vi "IGC100.vi"(8 "IGC100 B Error":refnum<vi>, 9 "IGC100 A Error":refnum<vi>, 11 "QUIT":refnum<vi>) -> ()   [LabVIEW 2018]
uses:
  <vilib>/Utility/error.llb/DialogType.ctl
  <vilib>/Analysis/baseanly.llb/Mean (DBL).vi
  <vilib>/Analysis/NI_AALBase.lvlib
panel:
  out "Main Error":errorcluster
  in  "IGC100":T1(tab)
  out "A PG1":dbl caption="PG1"
  out "A AN4":dbl caption="AN4"
  out "A AN3":dbl caption="AN3"
  out "A AN2":dbl caption="AN2"
  out "A AN1":dbl caption="AN1"
  out "A CM4":dbl caption="CM4"
  out "A CM3":dbl caption="CM3"
  out "A CM2":dbl caption="CM2"
  out "A IG2":dbl caption="IG2" format="%#_4e"
  out "A IG1":dbl caption="IG1" format="%#_4e"
  out "A PG2":dbl caption="PG2"
  out "A CM1":dbl caption="CM1"
  out "IGC100 B Status":string
  out "IGC100 A Status":string
  out "B IG1":dbl caption="IG1" format="%#2_4e"
  out "B IG2":dbl caption="IG2"
  out "B PG1":dbl caption="PG1" format="%#2_4e"
  out "B PG2":dbl caption="PG2" format="%#_4e"
  out "B AN1":dbl caption="AN1"
  out "B AN2":dbl caption="AN2"
  out "B AN3":dbl caption="AN3"
  out "B AN4":dbl caption="AN4"
  out "B CM1":dbl caption="CM1"
  out "B CM2":dbl caption="CM2"
  out "B CM3":dbl caption="CM3"
  out "B CM4":dbl caption="CM4"
  out "Logging":bool
  in  "Log Pressures":bool
  in  "Advanced Settings":bool caption="(This may take some\ntime to load.)"
  in  "Communication Interval (ms)":u32
  in  "Log Interval (s)":u32=1 min=1
  in  "Averaging Time (s)":u32=1
  in  "Enable IGC100 A":bool=TRUE
  in  "Enable IGC100 B":bool=TRUE
  out "IGC100 B Online":bool
  out "IGC100 A Online":bool
  in  "IGC100 A Port":refnum<visa-resource-name>="COM11"
  in  "IGC100 B Port":refnum<visa-resource-name>="COM9"
  out "IGC100 A error":errorcluster
  out "IGC100 B error":errorcluster
  # "IG1"
  # "IGC100 A"
  # "IGC100 B"
  # "Units are in Torr"
  # "Measurements continue after window is closed."
  # "Turn off the logging feature to save CPU power and\nhard drive space."
  # "Currenty, the first column in the log file is the time of day, in hours, expressed as a decmal.  The 24 measurements then follow in the order specified in the IGC100 manual.  First for A (12), then B (another 12).\n\nIG1, IG2, PG1,... AN4"
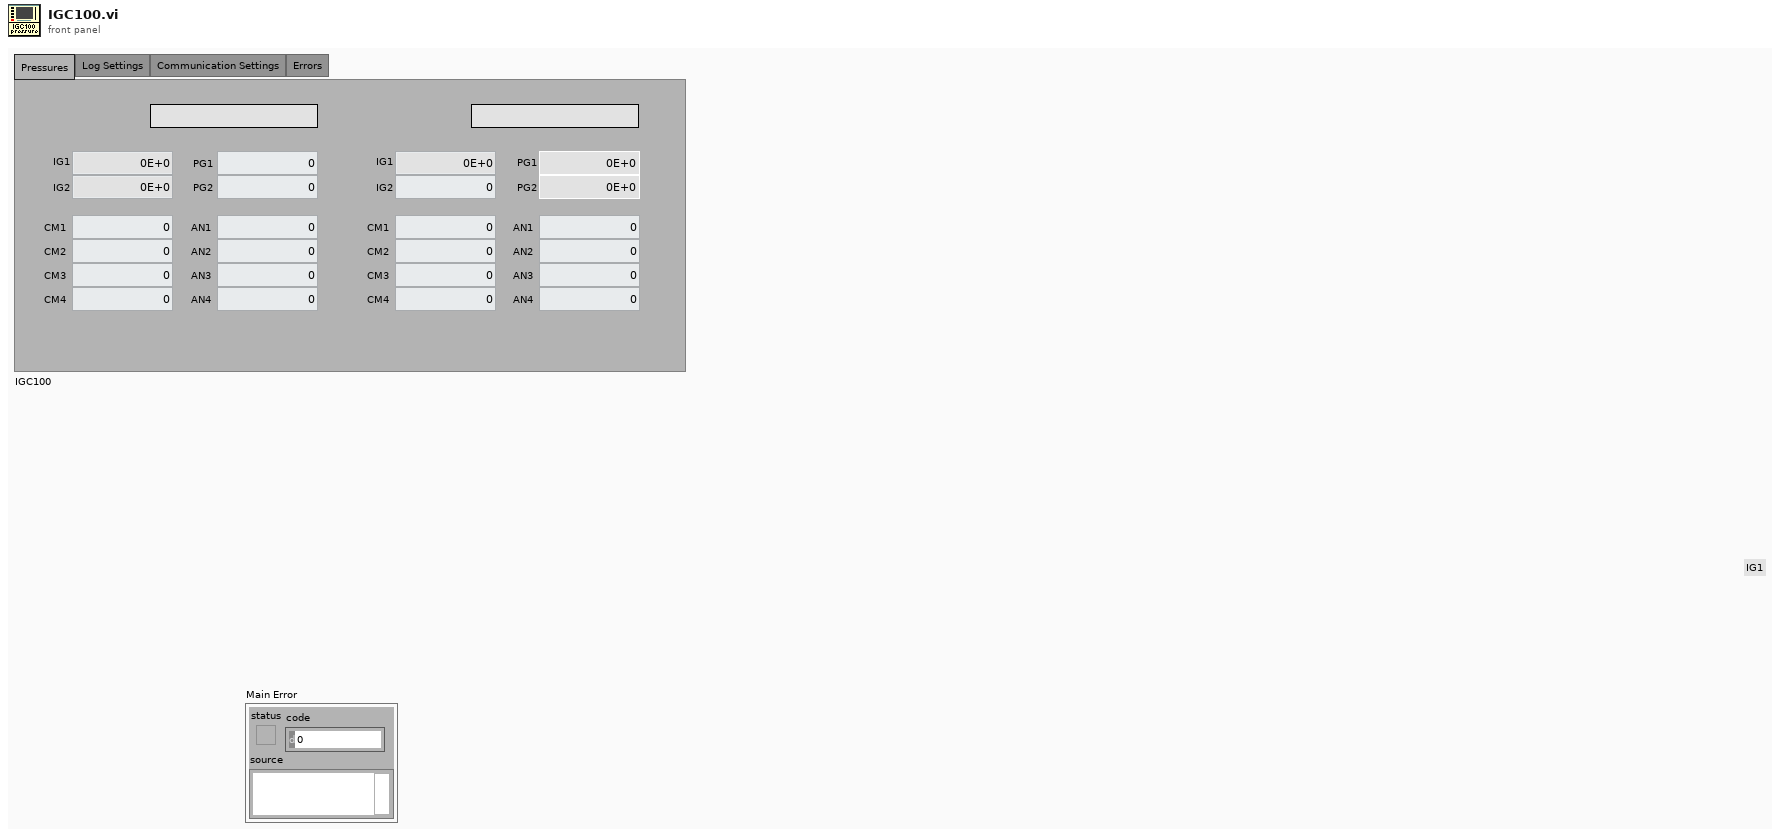
[diagram p1: front panel]
types:
  T1 = enum32{"Pressures", "Log Settings", "Communication Settings", "Errors"}
  T2 = typedef "DialogType.ctl" = u16
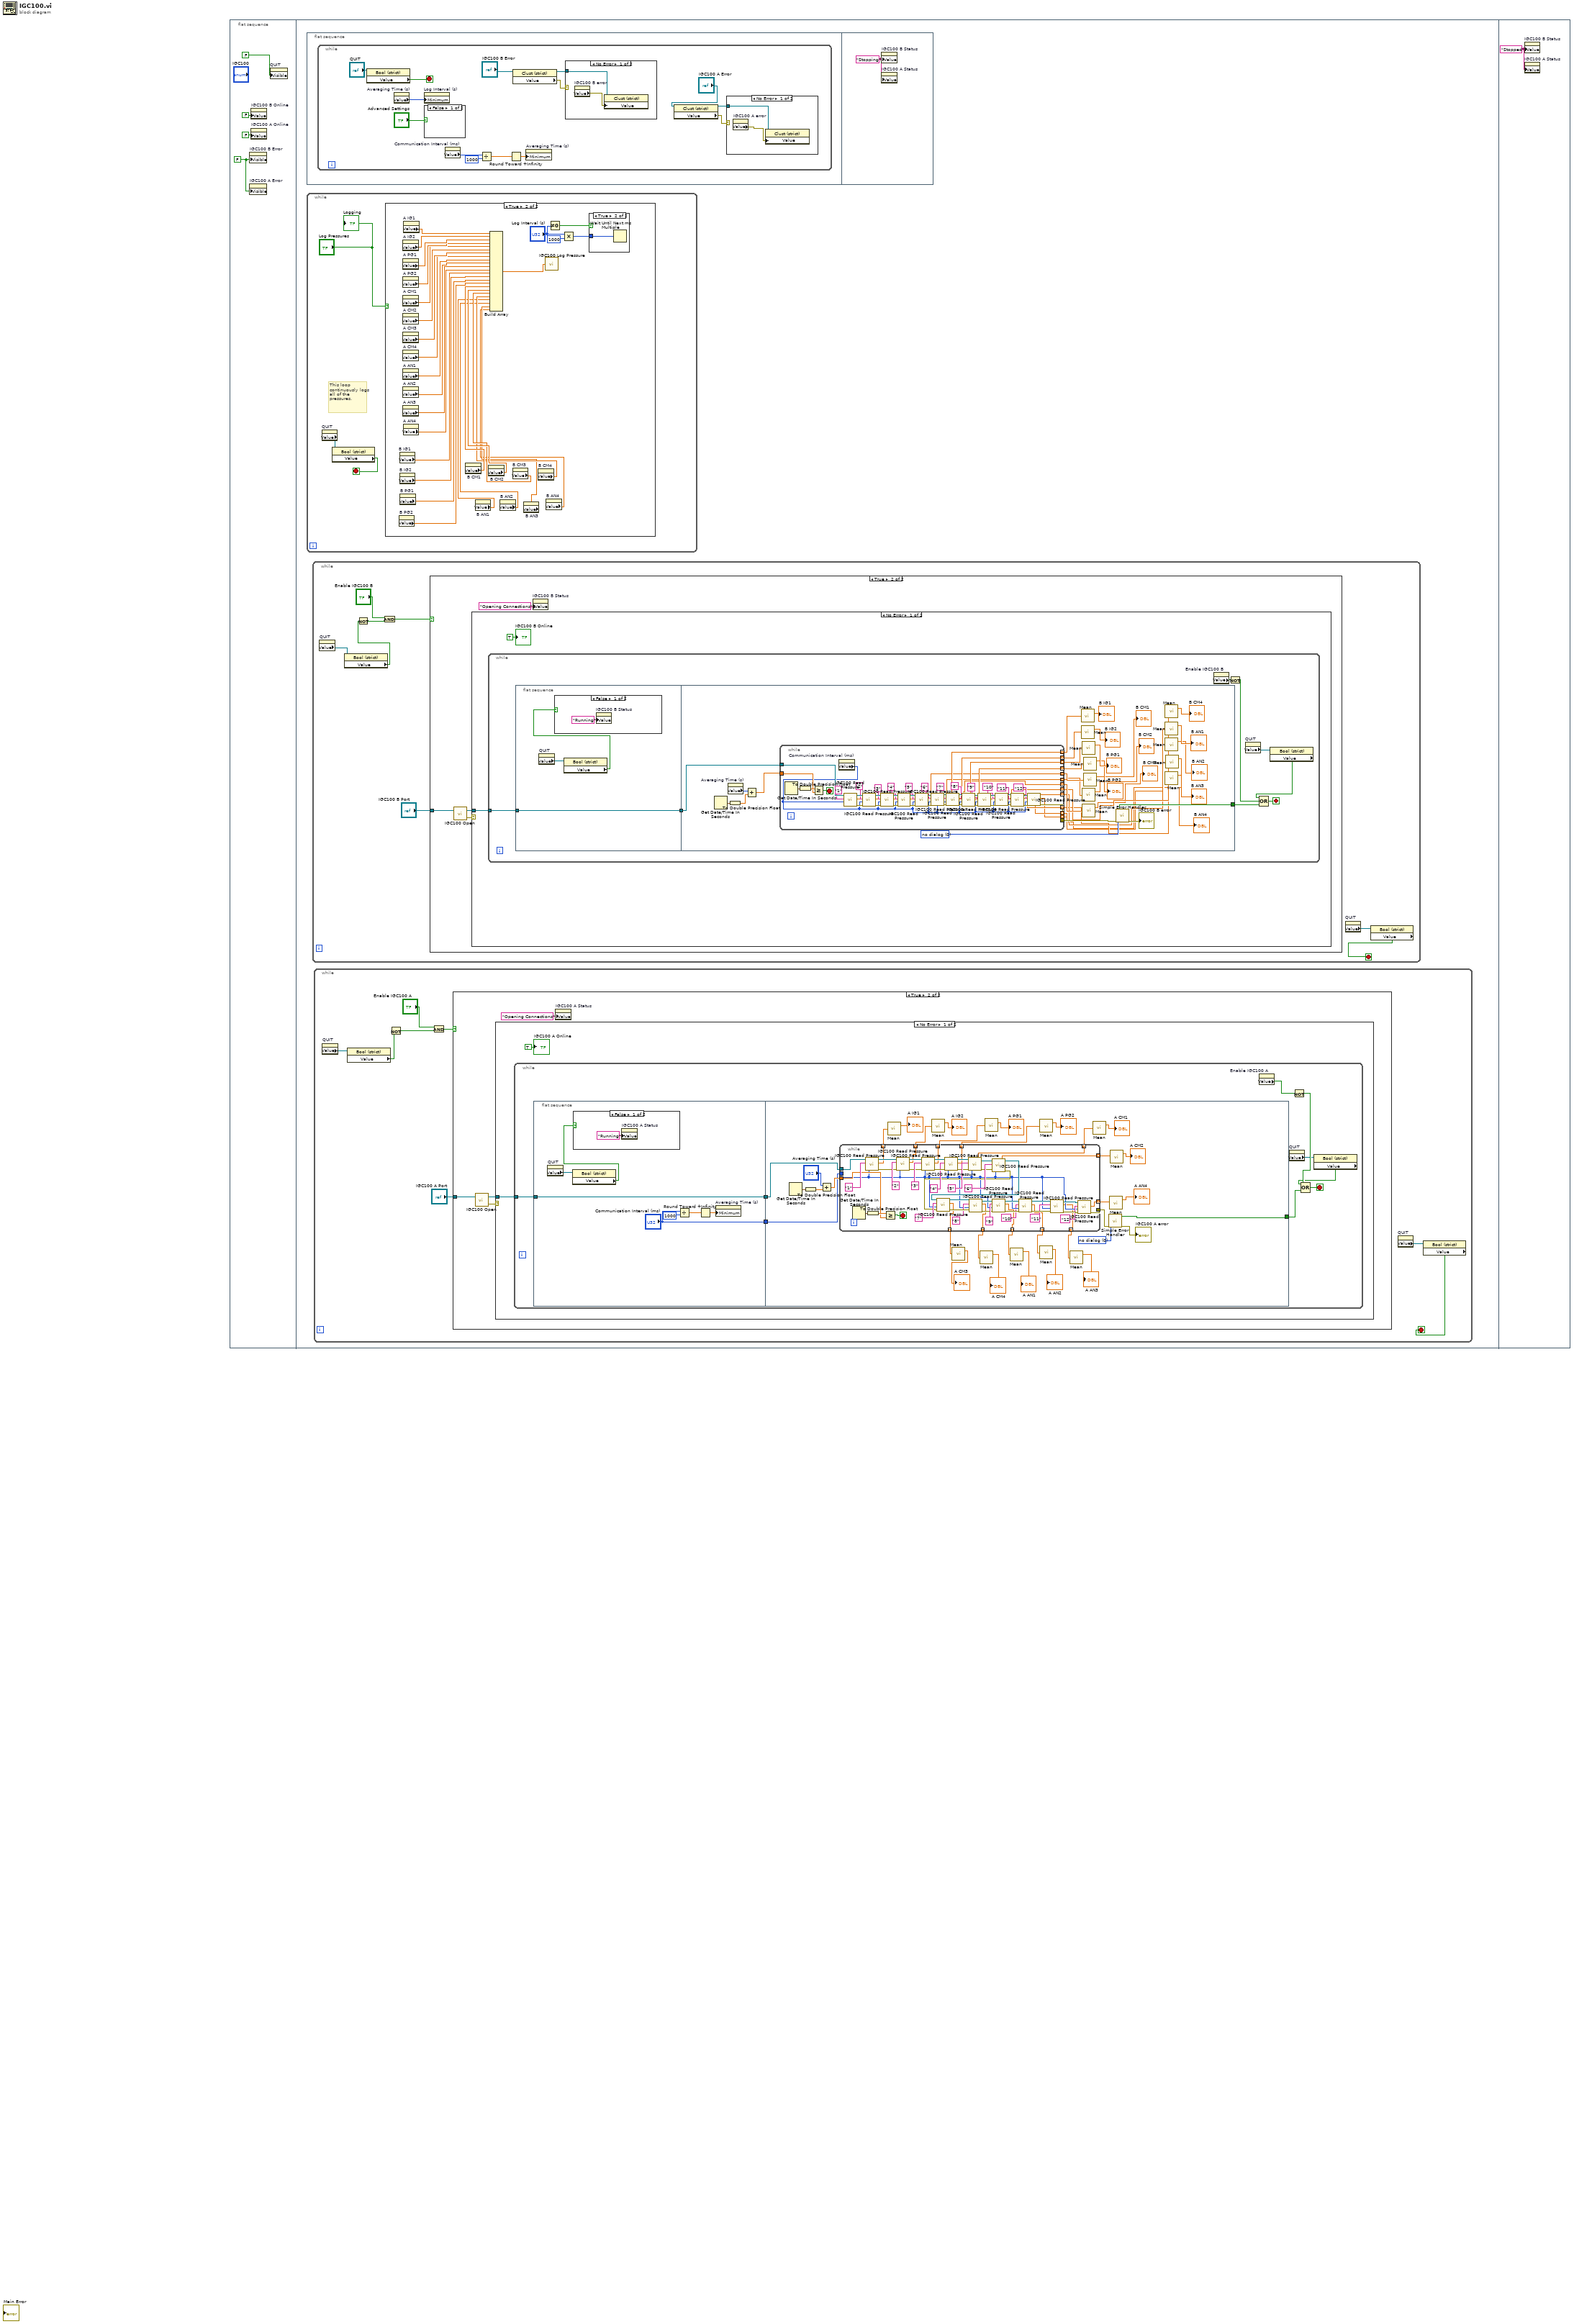
[diagram p0: block diagram]
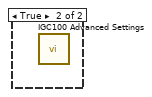
[diagram p4: hidden frame]
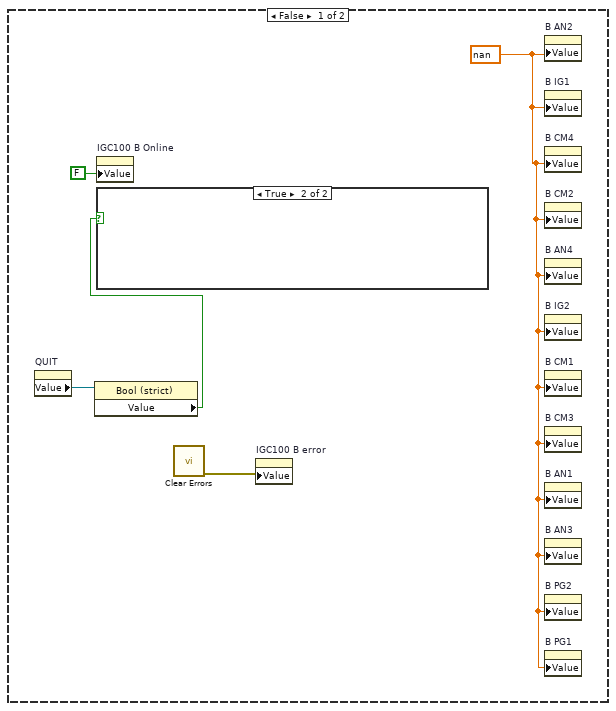
[diagram p7: hidden frame]
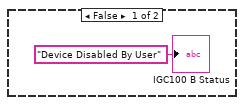
[diagram p8: hidden frame]
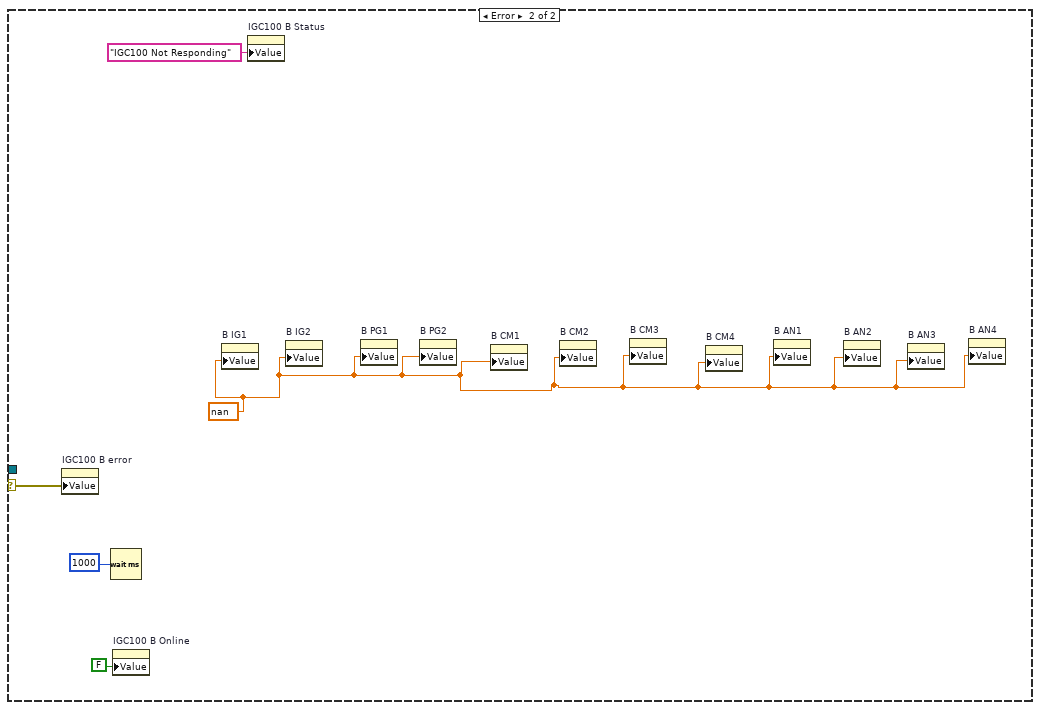
[diagram p10: hidden frame]
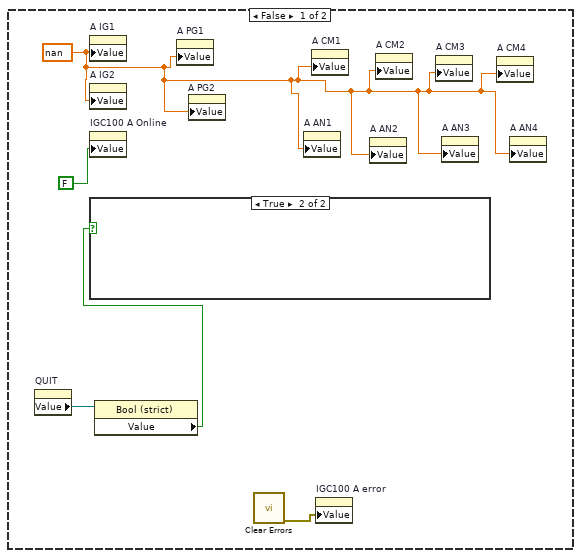
[diagram p11: hidden frame]
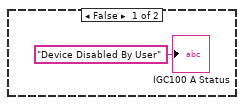
[diagram p12: hidden frame]
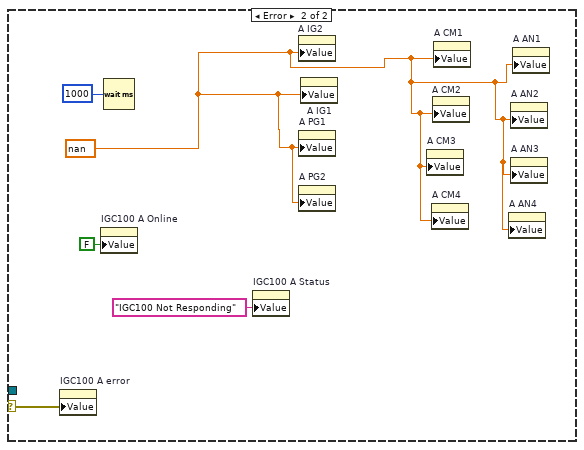
[diagram p14: hidden frame]
diagram:
  n1 = flat-sequence {
    frame #0 {
      w1 = FALSE ("Visible")
      n2 = property on="IGC100 B Error" class="LVObjRef (strict)"("Visible"=w1) -> ()  [unwired: 2 in, 2 out]
      n3 = property on="IGC100 A Error" class="LVObjRef (strict)"("Visible"=w1) -> ()  [unwired: 2 in, 2 out]
      n4 = property on="IGC100 B Online" class="Bool (strict)"("Value"=FALSE ("IGC100 Prep Online")) -> ()  [unwired: 2 in, 2 out]
      n5 = property on="IGC100 A Online" class="Bool (strict)"("Value"=FALSE ("IGC100 Main Online")) -> ()  [unwired: 2 in, 2 out]
      n6 = property on="QUIT" class="LVObjRef (strict)"("Visible"=FALSE ("QUIT")) -> ()  [unwired: 2 in, 2 out]
    }
    frame #1 {
      n7 = flat-sequence {
        frame #0 {
          n8 = while {
            stop <- w17 stop-if-true
            n9 = property on="Property Node" class="Bool (strict)"(reference="QUIT") -> ("Value"=w17:bool)  [unwired: 1 in, 2 out]
            n10 = property on="Averaging Time (s)" class="DigNum (strict)"() -> ("Value"=w12:u32)  [unwired: 2 in, 2 out]
            n11 = property on="Log Interval (s)" class="DigNum (strict)"("Minimum"=w12) -> ()  [unwired: 2 in, 2 out]
            n12 = case shown="False" "Advanced Settings" {
              frame False {
              }
              frame True {
                n13 = call "IGC100 Advanced Settings.vi"() -> ()  [unwired: 12 in]
              }
            }
            n14 = property on="Communication Interval (ms)" class="DigNum (strict)"() -> ("Value"=w14:u32)  [unwired: 2 in, 2 out]
            n15 = Divide(x=w14, y=u32 1000) -> (x/y=w15:dbl)
            n16 = Round Toward +Infinity(x=w15) -> (ceil(x): smallest int >= x=w16:dbl)
            n17 = property on="Property Node" class="Clust (strict)"(reference="IGC100 B Error") -> (reference out=w8:refnum<vi>, "Value"=w9:errorcluster)  [unwired: 1 in, 1 out]
            n18 = property on="Averaging Time (s)" class="DigNum (strict)"("Minimum"=w16) -> ()  [unwired: 2 in, 2 out]
            n19 = case shown="No Error" w9 {
              tunnel: w8 -> [w21 _]
              frame No Error {
                n20 = property on="IGC100 B error" class="Clust (strict)"() -> ("Value"=w22:errorcluster)  [unwired: 2 in, 2 out]
                n21 = property on="Property Node" class="Clust (strict)"(reference=w21, "Value"=w22) -> ()  [unwired: 1 in, 2 out]
              }
              frame Error {
              }
            }
            n22 = property on="Property Node" class="Clust (strict)"(reference="IGC100 A Error") -> (reference out=w7:refnum<vi>, "Value"=w6:errorcluster)  [unwired: 1 in, 1 out]
            n23 = case shown="No Error" w6 {
              tunnel: w7 -> [w20 _]
              frame No Error {
                n24 = property on="IGC100 A error" class="Clust (strict)"() -> ("Value"=w19:errorcluster)  [unwired: 2 in, 2 out]
                n25 = property on="Property Node" class="Clust (strict)"(reference=w20, "Value"=w19) -> ()  [unwired: 1 in, 2 out]
              }
              frame Error {
              }
            }
          }
        }
        frame #1 {
          w23 = "Stopping" ("IGC100 Main Status")
          n26 = property on="IGC100 B Status" class="Str"("Value"=w23) -> ()  [unwired: 2 in, 2 out]
          n27 = property on="IGC100 A Status" class="Str"("Value"=w23) -> ()  [unwired: 2 in, 2 out]
        }
      }
      n28 = while {
        stop <- w25 stop-if-true
        # "This loop continuously logs all of the pressures."
        n29 = property on="QUIT" class="LVObjRef (strict)"() -> ("Value"=w26:refnum<vi>)  [unwired: 2 in, 2 out]
        n30 = property on="Property Node" class="Bool (strict)"(reference=w26) -> ("Value"=w25:bool)  [unwired: 1 in, 2 out]
        n31 = case shown="True" "Log Pressures" {
          frame False {
          }
          frame True {
            n32 = property on="B PG2" class="DigNum (strict)"() -> ("Value"=w36:dbl)  [unwired: 2 in, 2 out]
            n33 = property on="B IG1" class="DigNum (strict)"() -> ("Value"=w39:dbl)  [unwired: 2 in, 2 out]
            n34 = property on="B IG2" class="DigNum (strict)"() -> ("Value"=w38:dbl)  [unwired: 2 in, 2 out]
            n35 = property on="B PG1" class="DigNum (strict)"() -> ("Value"=w37:dbl)  [unwired: 2 in, 2 out]
            n36 = property on="A IG2" class="DigNum (strict)"() -> ("Value"=w50:dbl)  [unwired: 2 in, 2 out]
            n37 = property on="A PG1" class="DigNum (strict)"() -> ("Value"=w49:dbl)  [unwired: 2 in, 2 out]
            n38 = property on="A PG2" class="DigNum (strict)"() -> ("Value"=w48:dbl)  [unwired: 2 in, 2 out]
            n39 = property on="A CM1" class="DigNum (strict)"() -> ("Value"=w47:dbl)  [unwired: 2 in, 2 out]
            n40 = property on="A CM2" class="DigNum (strict)"() -> ("Value"=w46:dbl)  [unwired: 2 in, 2 out]
            n41 = property on="A CM3" class="DigNum (strict)"() -> ("Value"=w45:dbl)  [unwired: 2 in, 2 out]
            n42 = property on="A CM4" class="DigNum (strict)"() -> ("Value"=w44:dbl)  [unwired: 2 in, 2 out]
            n43 = property on="A AN1" class="DigNum (strict)"() -> ("Value"=w43:dbl)  [unwired: 2 in, 2 out]
            n44 = property on="A AN2" class="DigNum (strict)"() -> ("Value"=w42:dbl)  [unwired: 2 in, 2 out]
            n45 = property on="A AN3" class="DigNum (strict)"() -> ("Value"=w41:dbl)  [unwired: 2 in, 2 out]
            n46 = property on="A AN4" class="DigNum (strict)"() -> ("Value"=w40:dbl)  [unwired: 2 in, 2 out]
            n47 = property on="A IG1" class="DigNum (strict)"() -> ("Value"=w51:dbl)  [unwired: 2 in, 2 out]
            n48 = property on="B CM1" class="DigNum (strict)"() -> ("Value"=w35:dbl)  [unwired: 2 in, 2 out]
            n49 = property on="B AN1" class="DigNum (strict)"() -> ("Value"=w31:dbl)  [unwired: 2 in, 2 out]
            n50 = property on="B CM2" class="DigNum (strict)"() -> ("Value"=w34:dbl)  [unwired: 2 in, 2 out]
            n51 = property on="B AN2" class="DigNum (strict)"() -> ("Value"=w30:dbl)  [unwired: 2 in, 2 out]
            n52 = property on="B CM3" class="DigNum (strict)"() -> ("Value"=w33:dbl)  [unwired: 2 in, 2 out]
            n53 = property on="B AN3" class="DigNum (strict)"() -> ("Value"=w29:dbl)  [unwired: 2 in, 2 out]
            n54 = property on="B CM4" class="DigNum (strict)"() -> ("Value"=w32:dbl)  [unwired: 2 in, 2 out]
            n55 = property on="B AN4" class="DigNum (strict)"() -> ("Value"=w28:dbl)  [unwired: 2 in, 2 out]
            n56 = Build Array(w51, w50, w49, w48, w47, w46, w45, w44, w43, w42, w41, w40, w39, w38, w37, w36, w35, w34, w33, w32, w31, w30, w29, w28) -> (w27:dbl[])
            n57 = call "IGC100 Log Pressure.vi"("Array"=w27) -> ()
            n58 = Not Equal To 0?(x="Log Interval (s)") -> (x != 0?=w55:bool)
            n59 = Multiply(x="Log Interval (s)", y=u32 1000) -> (x*y=w52:u32)
            n60 = case shown="True" w55 {
              tunnel: w52 -> [_ w56]
              frame False {
              }
              frame True {
                n61 = Wait Until Next ms Multiple(millisecond multiple=w56) -> ()  [unwired: 1 out]
              }
            }
          }
        }
        "Logging" <- "Log Pressures"
      }
      n62 = while {
        stop <- w57 stop-if-true
        n63 = property on="QUIT" class="LVObjRef (strict)"() -> ("Value"=w60:refnum<vi>)  [unwired: 2 in, 2 out]
        n64 = property on="Property Node" class="Bool (strict)"(reference=w60) -> ("Value"=w59:bool)  [unwired: 1 in, 2 out]
        n65 = Not(x=w59) -> (.not. x?=w61:bool)
        n66 = And(x="Enable IGC100 B", y=w61) -> (x .and. y?=w63:bool)
        n67 = case shown="True" w63 {
          tunnel: "IGC100 B Port" -> [_ w74]
          frame False {
            w65 = nan ("Prep Chamber Ion")
            n68 = property on="QUIT" class="LVObjRef (strict)"() -> ("Value"=w68:refnum<vi>)  [unwired: 2 in, 2 out]
            n69 = property on="Property Node" class="Bool (strict)"(reference=w68) -> ("Value"=w67:bool)  [unwired: 1 in, 2 out]
            n70 = property on="IGC100 B Online" class="Bool (strict)"("Value"=FALSE ("IGC100 Prep Online")) -> ()  [unwired: 2 in, 2 out]
            n71 = case shown="True" w67 {
              frame False {
                "IGC100 B Status" <- "Device Disabled By User" ("IGC100 Main Status")
              }
              frame True {
              }
            }
            n72 = call <vilib>:"Clear Errors.vi"() -> ("error out"=w66:errorcluster)  [unwired: 6 in, 1 out]
            n73 = property on="IGC100 B error" class="Clust (strict)"("Value"=w66) -> ()  [unwired: 2 in, 2 out]
            n74 = property on="B AN2" class="DigNum (strict)"("Value"=w65) -> ()  [unwired: 2 in, 2 out]
            n75 = property on="B IG1" class="DigNum (strict)"("Value"=w65) -> ()  [unwired: 2 in, 2 out]
            n76 = property on="B CM4" class="DigNum (strict)"("Value"=w65) -> ()  [unwired: 2 in, 2 out]
            n77 = property on="B CM2" class="DigNum (strict)"("Value"=w65) -> ()  [unwired: 2 in, 2 out]
            n78 = property on="B AN4" class="DigNum (strict)"("Value"=w65) -> ()  [unwired: 2 in, 2 out]
            n79 = property on="B IG2" class="DigNum (strict)"("Value"=w65) -> ()  [unwired: 2 in, 2 out]
            n80 = property on="B CM1" class="DigNum (strict)"("Value"=w65) -> ()  [unwired: 2 in, 2 out]
            n81 = property on="B CM3" class="DigNum (strict)"("Value"=w65) -> ()  [unwired: 2 in, 2 out]
            n82 = property on="B AN1" class="DigNum (strict)"("Value"=w65) -> ()  [unwired: 2 in, 2 out]
            n83 = property on="B AN3" class="DigNum (strict)"("Value"=w65) -> ()  [unwired: 2 in, 2 out]
            n84 = property on="B PG2" class="DigNum (strict)"("Value"=w65) -> ()  [unwired: 2 in, 2 out]
            n85 = property on="B PG1" class="DigNum (strict)"("Value"=w65) -> ()  [unwired: 2 in, 2 out]
          }
          frame True {
            n86 = call "IGC100 Open.vi"("VISA in"=w74) -> ("error out"=w72:errorcluster, "VISA out"=w73:refnum<visa-resource-name>)  [unwired: 1 in]
            n87 = case shown="No Error" w72 {
              selector: w72 -> [_ w177]
              tunnel: w73 -> [w76 _]
              frame No Error {
                n88 = while {
                  tunnel: w76 -> [w84]
                  stop <- w81 stop-if-true
                  n89 = flat-sequence {
                    tunnel: w84 -> [w87]
                    tunnel: [w87] -> w79
                    tunnel: [w116] -> w80
                    tunnel: w79 -> [w121]
                    frame #0 {
                      n90 = property on="QUIT" class="LVObjRef (strict)"() -> ("Value"=w86:refnum<vi>)  [unwired: 2 in, 2 out]
                      n91 = property on="Property Node" class="Bool (strict)"(reference=w86) -> ("Value"=w85:bool)  [unwired: 1 in, 2 out]
                      n92 = case shown="False" w85 {
                        frame False {
                          n93 = property on="IGC100 B Status" class="Str"("Value"="Running" ("IGC100 Main Status")) -> ()  [unwired: 2 in, 2 out]
                        }
                        frame True {
                        }
                      }
                    }
                    frame #1 {
                      w113 = T2 0 items=["no dialog", "OK message", "continue or stop message", "OK message + warnings", "continue/stop + warnings"] ("type of dialog (OK msg:1)")
                      n94 = Get Date/Time In Seconds() -> (seconds since 1Jan1904=w120:timestamp)
                      n95 = property on="Averaging Time (s)" class="DigNum (strict)"() -> ("Value"=w115:u32)  [unwired: 2 in, 2 out]
                      n96 = To Double Precision Float(number=w120) -> (double precision float=w119:dbl)
                      n97 = Add(x=w115, y=w119) -> (x+y=w118:dbl)
                      n98 = while {
                        tunnel: w121 -> [w174]
                        tunnel: w118 -> [w170]
                        tunnel: [w146] -> w117
                        tunnel: [w133] -> w112 mode=indexing
                        tunnel: [w132] -> w110 mode=indexing
                        tunnel: [w131] -> w109 mode=indexing
                        tunnel: [w130] -> w108 mode=indexing
                        tunnel: [w129] -> w107 mode=indexing
                        tunnel: [w128] -> w106 mode=indexing
                        tunnel: [w127] -> w105 mode=indexing
                        tunnel: [w126] -> w104 mode=indexing
                        tunnel: [w125] -> w103 mode=indexing
                        tunnel: [w124] -> w102 mode=indexing
                        tunnel: [w123] -> w101 mode=indexing
                        tunnel: [w122] -> w100 mode=indexing
                        stop <- w163 stop-if-true
                        n99 = Get Date/Time In Seconds() -> (seconds since 1Jan1904=w172:timestamp)
                        n100 = To Double Precision Float(number=w172) -> (double precision float=w171:dbl)
                        n101 = Greater Or Equal?(x=w171, y=w170) -> (x >= y?=w163:bool)
                        n102 = property on="Communication Interval (ms)" class="DigNum (strict)"() -> ("Value"=w134:u32)  [unwired: 2 in, 2 out]
                        n103 = call "IGC100 Read Pressure.vi"("Communication Interval (ms)"=w134, "Channel"="1", "VISA in"=w174) -> ("error out"=w165:errorcluster, "Pressure"=w133:dbl, "VISA out"=w169:refnum<visa-resource-name>)  [unwired: 2 in]
                        n104 = call "IGC100 Read Pressure.vi"("error in"=w165, "Communication Interval (ms)"=w134, "Channel"="2", "VISA in"=w169) -> ("error out"=w164:errorcluster, "Pressure"=w132:dbl, "VISA out"=w168:refnum<visa-resource-name>)  [unwired: 1 in]
                        n105 = call "IGC100 Read Pressure.vi"("error in"=w164, "Communication Interval (ms)"=w134, "Channel"="3", "VISA in"=w168) -> ("error out"=w161:errorcluster, "Pressure"=w131:dbl, "VISA out"=w162:refnum<visa-resource-name>)  [unwired: 1 in]
                        n106 = call "IGC100 Read Pressure.vi"("error in"=w161, "Communication Interval (ms)"=w134, "Channel"="4", "VISA in"=w162) -> ("error out"=w153:errorcluster, "Pressure"=w130:dbl, "VISA out"=w160:refnum<visa-resource-name>)  [unwired: 1 in]
                        n107 = call "IGC100 Read Pressure.vi"("error in"=w153, "Communication Interval (ms)"=w134, "Channel"="5", "VISA in"=w160) -> ("error out"=w152:errorcluster, "Pressure"=w129:dbl, "VISA out"=w159:refnum<visa-resource-name>)  [unwired: 1 in]
                        n108 = call "IGC100 Read Pressure.vi"("error in"=w152, "Communication Interval (ms)"=w134, "Channel"="6", "VISA in"=w159) -> ("error out"=w151:errorcluster, "Pressure"=w128:dbl, "VISA out"=w158:refnum<visa-resource-name>)  [unwired: 1 in]
                        n109 = call "IGC100 Read Pressure.vi"("error in"=w151, "Communication Interval (ms)"=w134, "Channel"="7", "VISA in"=w158) -> ("error out"=w150:errorcluster, "Pressure"=w127:dbl, "VISA out"=w157:refnum<visa-resource-name>)  [unwired: 1 in]
                        n110 = call "IGC100 Read Pressure.vi"("error in"=w150, "Communication Interval (ms)"=w134, "Channel"="8", "VISA in"=w157) -> ("error out"=w149:errorcluster, "Pressure"=w126:dbl, "VISA out"=w156:refnum<visa-resource-name>)  [unwired: 1 in]
                        n111 = call "IGC100 Read Pressure.vi"("error in"=w149, "Communication Interval (ms)"=w134, "Channel"="9", "VISA in"=w156) -> ("error out"=w135:errorcluster, "Pressure"=w125:dbl, "VISA out"=w155:refnum<visa-resource-name>)  [unwired: 1 in]
                        n112 = call "IGC100 Read Pressure.vi"("error in"=w135, "Communication Interval (ms)"=w134, "Channel"="10", "VISA in"=w155) -> ("error out"=w148:errorcluster, "Pressure"=w124:dbl, "VISA out"=w154:refnum<visa-resource-name>)  [unwired: 1 in]
                        n113 = call "IGC100 Read Pressure.vi"("error in"=w148, "Communication Interval (ms)"=w134, "Channel"="11", "VISA in"=w154) -> ("error out"=w147:errorcluster, "Pressure"=w123:dbl, "VISA out"=w145:refnum<visa-resource-name>)  [unwired: 1 in]
                        n114 = call "IGC100 Read Pressure.vi"("error in"=w147, "Communication Interval (ms)"=w134, "Channel"="12", "VISA in"=w145) -> ("error out"=w146:errorcluster, "Pressure"=w122:dbl)  [unwired: 1 in, 1 out]
                      }
                      n115 = call-poly <vilib>:"Mean.vi"("X"=w112) -> ("mean"=→"B IG1":dbl)  [unwired: 1 out]
                      n116 = call-poly <vilib>:"Mean.vi"("X"=w110) -> ("mean"=→"B IG2":dbl)  [unwired: 1 out]
                      n117 = call-poly <vilib>:"Mean.vi"("X"=w109) -> ("mean"=→"B PG1":dbl)  [unwired: 1 out]
                      n118 = call-poly <vilib>:"Mean.vi"("X"=w106) -> ("mean"=→"B CM2":dbl)  [unwired: 1 out]
                      n119 = call-poly <vilib>:"Mean.vi"("X"=w105) -> ("mean"=→"B CM3":dbl)  [unwired: 1 out]
                      n120 = call-poly <vilib>:"Mean.vi"("X"=w108) -> ("mean"=→"B PG2":dbl)  [unwired: 1 out]
                      n121 = call-poly <vilib>:"Mean.vi"("X"=w107) -> ("mean"=→"B CM1":dbl)  [unwired: 1 out]
                      n122 = call <vilib>:"Simple Error Handler.vi"("type of dialog (OK msg:1)"=w113, "error in (no error)"=w117) -> ("error?"=w116:bool, "error out"=→"IGC100 B error":errorcluster)  [unwired: 3 in, 3 out]
                      n123 = call-poly <vilib>:"Mean.vi"("X"=w104) -> ("mean"=→"B CM4":dbl)  [unwired: 1 out]
                      n124 = call-poly <vilib>:"Mean.vi"("X"=w103) -> ("mean"=→"B AN1":dbl)  [unwired: 1 out]
                      n125 = call-poly <vilib>:"Mean.vi"("X"=w102) -> ("mean"=→"B AN2":dbl)  [unwired: 1 out]
                      n126 = call-poly <vilib>:"Mean.vi"("X"=w100) -> ("mean"=→"B AN4":dbl)  [unwired: 1 out]
                      n127 = call-poly <vilib>:"Mean.vi"("X"=w101) -> ("mean"=→"B AN3":dbl)  [unwired: 1 out]
                    }
                  }
                  n128 = property on="Enable IGC100 B" class="Bool (strict)"() -> ("Value"=w83:bool)  [unwired: 2 in, 2 out]
                  n129 = Not(x=w83) -> (.not. x?=w82:bool)
                  n130 = property on="QUIT" class="LVObjRef (strict)"() -> ("Value"=w78:refnum<vi>)  [unwired: 2 in, 2 out]
                  n131 = property on="Property Node" class="Bool (strict)"(reference=w78) -> ("Value"=w77:bool)  [unwired: 1 in, 2 out]
                  n132 = Compound Arithmetic op=OR(w77, w82, w80) -> (w81:bool)
                }
                "IGC100 B Online" <- TRUE ("IGC100 Prep Online")
              }
              frame Error {
                w175 = nan ("Prep Chamber Ion")
                n133 = property on="IGC100 B error" class="Clust (strict)"("Value"=w177) -> ()  [unwired: 2 in, 2 out]
                n134 = Wait (ms)(milliseconds to wait=u32 1000) -> ()  [unwired: 1 out]
                n135 = property on="IGC100 B Online" class="Bool (strict)"("Value"=FALSE ("IGC100 Prep Online")) -> ()  [unwired: 2 in, 2 out]
                n136 = property on="B IG1" class="DigNum (strict)"("Value"=w175) -> ()  [unwired: 2 in, 2 out]
                n137 = property on="IGC100 B Status" class="Str"("Value"="IGC100 Not Responding" ("IGC100 Main Status")) -> ()  [unwired: 2 in, 2 out]
                n138 = property on="B IG2" class="DigNum (strict)"("Value"=w175) -> ()  [unwired: 2 in, 2 out]
                n139 = property on="B PG1" class="DigNum (strict)"("Value"=w175) -> ()  [unwired: 2 in, 2 out]
                n140 = property on="B PG2" class="DigNum (strict)"("Value"=w175) -> ()  [unwired: 2 in, 2 out]
                n141 = property on="B CM1" class="DigNum (strict)"("Value"=w175) -> ()  [unwired: 2 in, 2 out]
                n142 = property on="B CM2" class="DigNum (strict)"("Value"=w175) -> ()  [unwired: 2 in, 2 out]
                n143 = property on="B CM3" class="DigNum (strict)"("Value"=w175) -> ()  [unwired: 2 in, 2 out]
                n144 = property on="B CM4" class="DigNum (strict)"("Value"=w175) -> ()  [unwired: 2 in, 2 out]
                n145 = property on="B AN1" class="DigNum (strict)"("Value"=w175) -> ()  [unwired: 2 in, 2 out]
                n146 = property on="B AN2" class="DigNum (strict)"("Value"=w175) -> ()  [unwired: 2 in, 2 out]
                n147 = property on="B AN3" class="DigNum (strict)"("Value"=w175) -> ()  [unwired: 2 in, 2 out]
                n148 = property on="B AN4" class="DigNum (strict)"("Value"=w175) -> ()  [unwired: 2 in, 2 out]
              }
            }
            n149 = property on="IGC100 B Status" class="Str"("Value"="Opening Connections" ("IGC100 Main Status")) -> ()  [unwired: 2 in, 2 out]
          }
        }
        n150 = property on="QUIT" class="LVObjRef (strict)"() -> ("Value"=w58:refnum<vi>)  [unwired: 2 in, 2 out]
        n151 = property on="Property Node" class="Bool (strict)"(reference=w58) -> ("Value"=w57:bool)  [unwired: 1 in, 2 out]
      }
      n152 = while {
        stop <- w180 stop-if-true
        n153 = property on="QUIT" class="LVObjRef (strict)"() -> ("Value"=w183:refnum<vi>)  [unwired: 2 in, 2 out]
        n154 = property on="Property Node" class="Bool (strict)"(reference=w183) -> ("Value"=w182:bool)  [unwired: 1 in, 2 out]
        n155 = Not(x=w182) -> (.not. x?=w184:bool)
        n156 = And(x="Enable IGC100 A", y=w184) -> (x .and. y?=w186:bool)
        n157 = case shown="True" w186 {
          tunnel: "IGC100 A Port" -> [_ w196]
          frame False {
            w188 = nan ("Main Chamber")
            n158 = property on="QUIT" class="LVObjRef (strict)"() -> ("Value"=w191:refnum<vi>)  [unwired: 2 in, 2 out]
            n159 = property on="A IG1" class="DigNum (strict)"("Value"=w188) -> ()  [unwired: 2 in, 2 out]
            n160 = property on="A IG2" class="DigNum (strict)"("Value"=w188) -> ()  [unwired: 2 in, 2 out]
            n161 = property on="IGC100 A Online" class="Bool (strict)"("Value"=FALSE ("IGC100 Main Online")) -> ()  [unwired: 2 in, 2 out]
            n162 = property on="Property Node" class="Bool (strict)"(reference=w191) -> ("Value"=w190:bool)  [unwired: 1 in, 2 out]
            n163 = case shown="True" w190 {
              frame False {
                "IGC100 A Status" <- "Device Disabled By User" ("IGC100 Main Status")
              }
              frame True {
              }
            }
            n164 = property on="A PG1" class="DigNum (strict)"("Value"=w188) -> ()  [unwired: 2 in, 2 out]
            n165 = property on="A PG2" class="DigNum (strict)"("Value"=w188) -> ()  [unwired: 2 in, 2 out]
            n166 = call <vilib>:"Clear Errors.vi"() -> ("error out"=w189:errorcluster)  [unwired: 6 in, 1 out]
            n167 = property on="A AN1" class="DigNum (strict)"("Value"=w188) -> ()  [unwired: 2 in, 2 out]
            n168 = property on="A CM1" class="DigNum (strict)"("Value"=w188) -> ()  [unwired: 2 in, 2 out]
            n169 = property on="IGC100 A error" class="Clust (strict)"("Value"=w189) -> ()  [unwired: 2 in, 2 out]
            n170 = property on="A AN2" class="DigNum (strict)"("Value"=w188) -> ()  [unwired: 2 in, 2 out]
            n171 = property on="A CM2" class="DigNum (strict)"("Value"=w188) -> ()  [unwired: 2 in, 2 out]
            n172 = property on="A CM3" class="DigNum (strict)"("Value"=w188) -> ()  [unwired: 2 in, 2 out]
            n173 = property on="A AN3" class="DigNum (strict)"("Value"=w188) -> ()  [unwired: 2 in, 2 out]
            n174 = property on="A CM4" class="DigNum (strict)"("Value"=w188) -> ()  [unwired: 2 in, 2 out]
            n175 = property on="A AN4" class="DigNum (strict)"("Value"=w188) -> ()  [unwired: 2 in, 2 out]
          }
          frame True {
            n176 = call "IGC100 Open.vi"("VISA in"=w196) -> ("error out"=w194:errorcluster, "VISA out"=w195:refnum<visa-resource-name>)  [unwired: 1 in]
            n177 = case shown="No Error" w194 {
              selector: w194 -> [_ w306]
              tunnel: w195 -> [w199 _]
              frame No Error {
                n178 = while {
                  tunnel: w199 -> [w208]
                  stop <- w207 stop-if-true
                  n179 = flat-sequence {
                    tunnel: w208 -> [w215]
                    tunnel: [w215] -> w205
                    tunnel: ["Communication Interval (ms)"] -> w204
                    tunnel: [w246] -> w206
                    tunnel: w205 -> [w250]
                    tunnel: w204 -> [w243]
                    frame #0 {
                      n180 = property on="QUIT" class="LVObjRef (strict)"() -> ("Value"=w210:refnum<vi>)  [unwired: 2 in, 2 out]
                      n181 = property on="Property Node" class="Bool (strict)"(reference=w210) -> ("Value"=w209:bool)  [unwired: 1 in, 2 out]
                      n182 = case shown="False" w209 {
                        frame False {
                          n183 = property on="IGC100 A Status" class="Str"("Value"="Running" ("IGC100 Main Status")) -> ()  [unwired: 2 in, 2 out]
                        }
                        frame True {
                        }
                      }
                      n184 = Divide(x="Communication Interval (ms)", y=u32 1000) -> (x/y=w213:dbl)
                      n185 = Round Toward +Infinity(x=w213) -> (ceil(x): smallest int >= x=w214:dbl)
                      n186 = property on="Averaging Time (s)" class="DigNum (strict)"("Minimum"=w214) -> ()  [unwired: 2 in, 2 out]
                    }
                    frame #1 {
                      w242 = T2 0 items=["no dialog", "OK message", "continue or stop message", "OK message + warnings", "continue/stop + warnings"] ("type of dialog (OK msg:1)")
                      n187 = Get Date/Time In Seconds() -> (seconds since 1Jan1904=w249:timestamp)
                      n188 = To Double Precision Float(number=w249) -> (double precision float=w248:dbl)
                      n189 = Add(x="Averaging Time (s)", y=w248) -> (x+y=w247:dbl)
                      n190 = while {
                        tunnel: w250 -> [w303]
                        tunnel: w247 -> [w299]
                        tunnel: w243 -> [w265]
                        tunnel: [w286] -> w241
                        tunnel: [w263] -> w240 mode=indexing
                        tunnel: [w262] -> w238 mode=indexing
                        tunnel: [w261] -> w236 mode=indexing
                        tunnel: [w260] -> w234 mode=indexing
                        tunnel: [w259] -> w232 mode=indexing
                        tunnel: [w258] -> w230 mode=indexing
                        tunnel: [w257] -> w228 mode=indexing
                        tunnel: [w255] -> w227 mode=indexing
                        tunnel: [w254] -> w226 mode=indexing
                        tunnel: [w253] -> w225 mode=indexing
                        tunnel: [w252] -> w224 mode=indexing
                        tunnel: [w251] -> w223 mode=indexing
                        stop <- w292 stop-if-true
                        n191 = Get Date/Time In Seconds() -> (seconds since 1Jan1904=w301:timestamp)
                        n192 = call "IGC100 Read Pressure.vi"("Communication Interval (ms)"=w265, "Channel"="1", "VISA in"=w303) -> ("error out"=w294:errorcluster, "Pressure"=w263:dbl, "VISA out"=w298:refnum<visa-resource-name>)  [unwired: 2 in]
                        n193 = To Double Precision Float(number=w301) -> (double precision float=w300:dbl)
                        n194 = Greater Or Equal?(x=w300, y=w299) -> (x >= y?=w292:bool)
                        n195 = call "IGC100 Read Pressure.vi"("error in"=w294, "Communication Interval (ms)"=w265, "Channel"="2", "VISA in"=w298) -> ("error out"=w293:errorcluster, "Pressure"=w262:dbl, "VISA out"=w297:refnum<visa-resource-name>)  [unwired: 1 in]
                        n196 = call "IGC100 Read Pressure.vi"("error in"=w293, "Communication Interval (ms)"=w265, "Channel"="3", "VISA in"=w297) -> ("error out"=w291:errorcluster, "Pressure"=w261:dbl, "VISA out"=w285:refnum<visa-resource-name>)  [unwired: 1 in]
                        n197 = call "IGC100 Read Pressure.vi"("error in"=w291, "Communication Interval (ms)"=w265, "Channel"="4", "VISA in"=w285) -> ("error out"=w268:errorcluster, "Pressure"=w260:dbl, "VISA out"=w284:refnum<visa-resource-name>)  [unwired: 1 in]
                        n198 = call "IGC100 Read Pressure.vi"("error in"=w268, "Communication Interval (ms)"=w265, "Channel"="5", "VISA in"=w284) -> ("error out"=w267:errorcluster, "Pressure"=w259:dbl, "VISA out"=w283:refnum<visa-resource-name>)  [unwired: 1 in]
                        n199 = call "IGC100 Read Pressure.vi"("error in"=w267, "Communication Interval (ms)"=w265, "Channel"="6", "VISA in"=w283) -> ("error out"=w266:errorcluster, "Pressure"=w258:dbl, "VISA out"=w282:refnum<visa-resource-name>)  [unwired: 1 in]
                        n200 = call "IGC100 Read Pressure.vi"("error in"=w266, "Communication Interval (ms)"=w265, "Channel"="7", "VISA in"=w282) -> ("error out"=w290:errorcluster, "Pressure"=w257:dbl, "VISA out"=w281:refnum<visa-resource-name>)  [unwired: 1 in]
                        n201 = call "IGC100 Read Pressure.vi"("error in"=w290, "Communication Interval (ms)"=w265, "Channel"="8", "VISA in"=w281) -> ("error out"=w256:errorcluster, "Pressure"=w255:dbl, "VISA out"=w280:refnum<visa-resource-name>)  [unwired: 1 in]
                        n202 = call "IGC100 Read Pressure.vi"("error in"=w256, "Communication Interval (ms)"=w265, "Channel"="9", "VISA in"=w280) -> ("error out"=w289:errorcluster, "Pressure"=w254:dbl, "VISA out"=w279:refnum<visa-resource-name>)  [unwired: 1 in]
                        n203 = call "IGC100 Read Pressure.vi"("error in"=w289, "Communication Interval (ms)"=w265, "Channel"="10", "VISA in"=w279) -> ("error out"=w288:errorcluster, "Pressure"=w253:dbl, "VISA out"=w278:refnum<visa-resource-name>)  [unwired: 1 in]
                        n204 = call "IGC100 Read Pressure.vi"("error in"=w288, "Communication Interval (ms)"=w265, "Channel"="11", "VISA in"=w278) -> ("error out"=w287:errorcluster, "Pressure"=w252:dbl, "VISA out"=w277:refnum<visa-resource-name>)  [unwired: 1 in]
                        n205 = call "IGC100 Read Pressure.vi"("error in"=w287, "Communication Interval (ms)"=w265, "Channel"="12", "VISA in"=w277) -> ("error out"=w286:errorcluster, "Pressure"=w251:dbl)  [unwired: 1 in, 1 out]
                      }
                      n206 = call-poly <vilib>:"Mean.vi"("X"=w240) -> ("mean"=→"A IG1":dbl)  [unwired: 1 out]
                      n207 = call-poly <vilib>:"Mean.vi"("X"=w238) -> ("mean"=→"A IG2":dbl)  [unwired: 1 out]
                      n208 = call-poly <vilib>:"Mean.vi"("X"=w228) -> ("mean"=→"A CM3":dbl)  [unwired: 1 out]
                      n209 = call-poly <vilib>:"Mean.vi"("X"=w227) -> ("mean"=→"A CM4":dbl)  [unwired: 1 out]
                      n210 = call-poly <vilib>:"Mean.vi"("X"=w236) -> ("mean"=→"A PG1":dbl)  [unwired: 1 out]
                      n211 = call-poly <vilib>:"Mean.vi"("X"=w226) -> ("mean"=→"A AN1":dbl)  [unwired: 1 out]
                      n212 = call-poly <vilib>:"Mean.vi"("X"=w234) -> ("mean"=→"A PG2":dbl)  [unwired: 1 out]
                      n213 = call-poly <vilib>:"Mean.vi"("X"=w225) -> ("mean"=→"A AN2":dbl)  [unwired: 1 out]
                      n214 = call-poly <vilib>:"Mean.vi"("X"=w224) -> ("mean"=→"A AN3":dbl)  [unwired: 1 out]
                      n215 = call-poly <vilib>:"Mean.vi"("X"=w232) -> ("mean"=→"A CM1":dbl)  [unwired: 1 out]
                      n216 = call <vilib>:"Simple Error Handler.vi"("type of dialog (OK msg:1)"=w242, "error in (no error)"=w241) -> ("error?"=w246:bool, "error out"=→"IGC100 A error":errorcluster)  [unwired: 3 in, 3 out]
                      n217 = call-poly <vilib>:"Mean.vi"("X"=w223) -> ("mean"=→"A AN4":dbl)  [unwired: 1 out]
                      n218 = call-poly <vilib>:"Mean.vi"("X"=w230) -> ("mean"=→"A CM2":dbl)  [unwired: 1 out]
                    }
                  }
                  n219 = property on="Enable IGC100 A" class="Bool (strict)"() -> ("Value"=w202:bool)  [unwired: 2 in, 2 out]
                  n220 = property on="QUIT" class="LVObjRef (strict)"() -> ("Value"=w201:refnum<vi>)  [unwired: 2 in, 2 out]
                  n221 = Not(x=w202) -> (.not. x?=w203:bool)
                  n222 = property on="Property Node" class="Bool (strict)"(reference=w201) -> ("Value"=w200:bool)  [unwired: 1 in, 2 out]
                  n223 = Compound Arithmetic op=OR(w200, w203, w206) -> (w207:bool)
                }
                "IGC100 A Online" <- TRUE ("IGC100 Main Online")
              }
              frame Error {
                w304 = nan ("Krypton")
                n224 = property on="IGC100 A error" class="Clust (strict)"("Value"=w306) -> ()  [unwired: 2 in, 2 out]
                n225 = property on="IGC100 A Online" class="Bool (strict)"("Value"=FALSE ("IGC100 Main Online")) -> ()  [unwired: 2 in, 2 out]
                n226 = Wait (ms)(milliseconds to wait=u32 1000) -> ()  [unwired: 1 out]
                n227 = property on="IGC100 A Status" class="Str"("Value"="IGC100 Not Responding" ("IGC100 Main Status")) -> ()  [unwired: 2 in, 2 out]
                n228 = property on="A IG2" class="DigNum (strict)"("Value"=w304) -> ()  [unwired: 2 in, 2 out]
                n229 = property on="A PG1" class="DigNum (strict)"("Value"=w304) -> ()  [unwired: 2 in, 2 out]
                n230 = property on="A PG2" class="DigNum (strict)"("Value"=w304) -> ()  [unwired: 2 in, 2 out]
                n231 = property on="A IG1" class="DigNum (strict)"("Value"=w304) -> ()  [unwired: 2 in, 2 out]
                n232 = property on="A CM3" class="DigNum (strict)"("Value"=w304) -> ()  [unwired: 2 in, 2 out]
                n233 = property on="A CM4" class="DigNum (strict)"("Value"=w304) -> ()  [unwired: 2 in, 2 out]
                n234 = property on="A CM2" class="DigNum (strict)"("Value"=w304) -> ()  [unwired: 2 in, 2 out]
                n235 = property on="A CM1" class="DigNum (strict)"("Value"=w304) -> ()  [unwired: 2 in, 2 out]
                n236 = property on="A AN4" class="DigNum (strict)"("Value"=w304) -> ()  [unwired: 2 in, 2 out]
                n237 = property on="A AN2" class="DigNum (strict)"("Value"=w304) -> ()  [unwired: 2 in, 2 out]
                n238 = property on="A AN3" class="DigNum (strict)"("Value"=w304) -> ()  [unwired: 2 in, 2 out]
                n239 = property on="A AN1" class="DigNum (strict)"("Value"=w304) -> ()  [unwired: 2 in, 2 out]
              }
            }
            n240 = property on="IGC100 A Status" class="Str"("Value"="Opening Connections" ("IGC100 Main Status")) -> ()  [unwired: 2 in, 2 out]
          }
        }
        n241 = property on="QUIT" class="LVObjRef (strict)"() -> ("Value"=w181:refnum<vi>)  [unwired: 2 in, 2 out]
        n242 = property on="Property Node" class="Bool (strict)"(reference=w181) -> ("Value"=w180:bool)  [unwired: 1 in, 2 out]
      }
    }
    frame #2 {
      w309 = "Stopped" ("IGC100 Main Status")
      n243 = property on="IGC100 B Status" class="Str"("Value"=w309) -> ()  [unwired: 2 in, 2 out]
      n244 = property on="IGC100 A Status" class="Str"("Value"=w309) -> ()  [unwired: 2 in, 2 out]
    }
  }
